vi "Input DMA Engine.vi"(10 "Parameters":variant, 11 "Process":refnum<class "Process.lvclass">) -> ()   [LabVIEW 2019, in "FPGA Addon Engine.lvlib"]
uses:
  FPGA Addon Engine.lvlib
  <vilib>/NI/NIVS Inline Async API/_VS Inline Async API/Process/Process.lvclass
  Types/DMA Input References.ctl
  <vilib>/NI VeriStand/Custom Device Waveform API/Multiple Waveforms Write (DBL)/Multiple Waveforms Write (DBL).lvclass
  Addon Shared/DMA Settings.ctl
  Addon Shared/Delacing Scheme.ctl
  Addon Shared/DMA Acquisition Mode.ctl
  Types/DMA Input Refs.ctl
  Addon Shared/Data Type.ctl
  <vilib>/NI/NIVS Inline Async API/_VS Inline Async API/Process/Process.lvclass/Process.ctl
  <vilib>/Platform/TimedLoop/XDataNode/timing_clust.ctl
  <vilib>/Platform/TimedLoop/XDataNode/nitl_modes.ctl
  <vilib>/Platform/TimedLoop/XDataNode/wakeup.ctl
  <vilib>/NI/NIVS Inline Async API/_Data Access Engine/Access Type Classes/Write/Write.lvclass/Write.ctl
  <vilib>/NI/NIVS Inline Async API/_Data Access Engine/Data Access Engine/Methods/Write.Data.vi
  <vilib>/NI/NIVS Inline Async API/_VS Inline Async API/Process/Data Member Access/Read Data Access.vi
  <vilib>/NI/NIVS Inline Async API/_Data Access Engine/Access Type Classes/Write/Write.ProcessData.vi
  <vilib>/NI/NIVS Inline Async API/_VS Inline Async API/Error Handling Process/SubVIs/Error.ConvertArray.vi
  <vilib>/NI/NIVS Inline Async API/_Data Access Engine/Access Type Classes/Write/Write.Buffer.vi
  <vilib>/NI/NIVS Inline Async API/_Data Access Engine/Access Type Classes/Write/Write.Commit.vi
  <vilib>/Utility/SystemLogging/Write to System Log.vi
  <vilib>/NI/NIVS Inline Async API/_Data Access Engine/Data Access Engine/Methods/Write.Lookup.vi
  <vilib>/FPGAPlugInAG/Dynamic/niLvFpga_Close_Dynamic.vi
  <vilib>/NI VeriStand/Custom Device Waveform API/Multiple Waveforms Write (DBL)/NI VeriStand - Close Multiple Waveforms Write Session (DBL).vi
  <vilib>/NI/NIVS Inline Async API/_Data Access Engine/Data Access Engine/Data Access Engine.lvclass
  <vilib>/Platform/TimedLoop/XDataNode/XDataNode.xnode
  <vilib>/rvi/interface/nirviCloseFPGA/nirviCloseFPGA.xnode
  <vilib>/NI VeriStand/Custom Device Waveform API/NI_VS Custom Device Waveform API.lvlib
  <vilib>/Platform/TimedLoop/XDataNode/XDNodeRunTimeDep.lvlib
  Addon Shared/FPGA Addon Shared.lvlib
panel:
  out "error out":errorcluster
  in  "error in (no error)":errorcluster
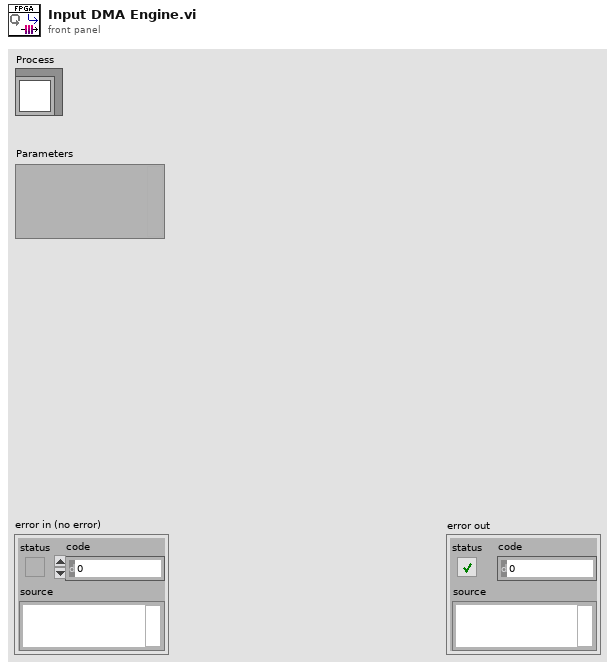
[diagram p1: front panel]
types:
  T1 = typedef "FPGA Addon Engine.lvlib/DMA Input References.ctl" = cluster{"Addon Name":string, "Waveform Ref":refnum<class "Multiple Waveforms Write (DBL).lvclass">, "DMA Name":string, "DMA Settings":T2, "Refs":T5}
  T2 = typedef "FPGA Addon Shared.lvlib/DMA Settings.ctl" = cluster{"Number of Channels":u8, "Delacing Scheme":T3, "Update Rate":u32, "dt":dbl, "Mode":T4, "Number of Samples":u32, "DMA Host Buffer":u32}
  T3 = typedef "FPGA Addon Shared.lvlib/Delacing Scheme.ctl" = enum8{"Interleaved", "Bitpacked"}
  T4 = typedef "FPGA Addon Shared.lvlib/DMA Acquisition Mode.ctl" = enum8{"Continuous", "Triggered Finite"}
  T5 = typedef "FPGA Addon Engine.lvlib/DMA Input Refs.ctl" = cluster{"Data Type":T6, "DMA_SGL":refnum<k20>, "DMA_U64":refnum<k20>, "DMA_I64":refnum<k20>, "DMA_FXP+/-32.8":refnum<k20>, "DMA_FXP+/-64.32":refnum<k20>, "DMA_U32":refnum<k20>, "DMA_U16":refnum<k20>, "DMA_U8":refnum<k20>, "DMA_I32":refnum<k20>, "DMA_I16":refnum<k20>, "DMA_I8":refnum<k20>, "DMA_FXP+/-32.16":refnum<k20>}
  T6 = typedef "FPGA Addon Shared.lvlib/Data Type.ctl" = enum8{"<Null>", "I8", "I16", "I32", "I64", "U8", "U16", "U32", "U64", "SGL", "Boolean", "Analog PWM In Settings", "Analog PWM In", "Digital PWM In Settings", "Digital PWM In", "Digital PWM Out", "Sine Out", "FXP+/-24.5", "FXP+/-16.5", "FXP+/-32.8", "FXP+/-64.32", "FXP+/-16.7", "FXP+/-20.5", "FXP+/-27.5", "FXP+/-32.16", "FXP +16.3", "FXP +18.3", "Digital Static In", "Digital Static Out", "Digital Static In Settings", "Digital WSS Out", "Quad Encoder Settings", "Quad Encoder In"}
  T7 = typedef "Data Access Engine.lvlib/Data Access Engine.lvclass/Write.DVR.ctl" = refnum<data-value>
  T8 = typedef "XDNodeRunTimeDep.lvlib/timing_clust.ctl" = cluster{"Expected End [f-1]":u64, "Actual End [f-1]":u64, "Finished Late? [f-1]":bool, "Expected End [i-1]":u64, "Actual End [i-1]":u64, "Finished Late? [i-1]":bool, "Expected Start [i]":u64, "Actual Start [i]":u64, "Expected Start [f]":u64, "Actual Start [f]":u64, "Source Name":string, "Structure Name":string, "Period":i64, "Deadline":i64, "Offset":i64, "Start":i64, "Priority":i32, "Timeout":i32, "Mode":T9, "Wakeup Reason":T10, "Error":errorcluster, "Source Type":string, "Secondary Source Type":string, "Global End Time":u64, "Global Start Time":u64, "Frame Duration":u64, "Iteration Duration":u64, "Assigned CPU":i32, "I/O Scan Engine Mode":u32}
  T9 = typedef "XDNodeRunTimeDep.lvlib/nitl_modes.ctl" = enum32{"No Change", "Process missed periods, maintain original phase", "Discard missed periods, maintain original phase", "Process missed periods, ignore original phase", "Discard missed periods, ignore original phase"}
  T10 = typedef "XDNodeRunTimeDep.lvlib/wakeup.ctl" = enum32{"Normal", "Aborted", "Asynchronous wakeup", "Timing source error", "Timed loop error", "Timeout"}
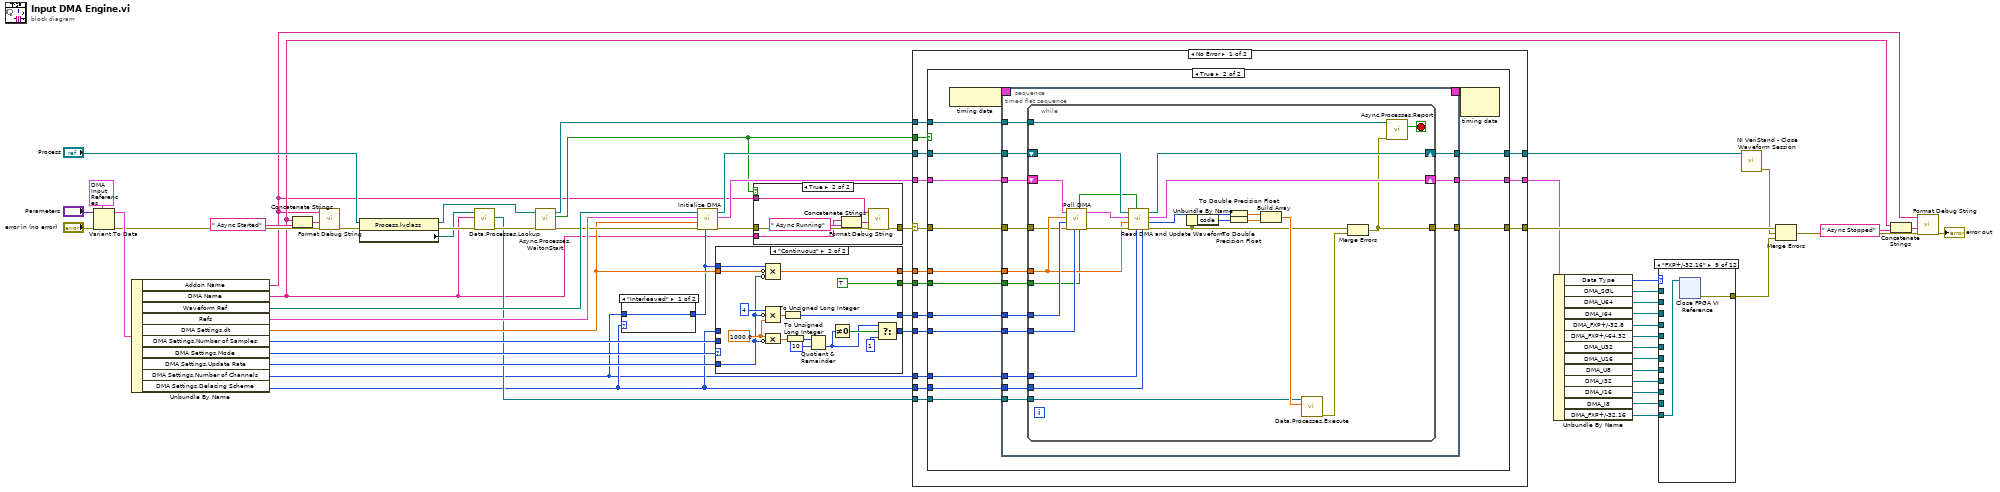
[diagram p0: block diagram]
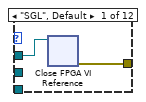
[diagram p2: hidden frame]
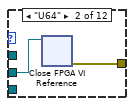
[diagram p3: hidden frame]
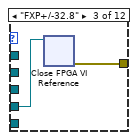
[diagram p4: hidden frame]
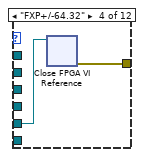
[diagram p5: hidden frame]
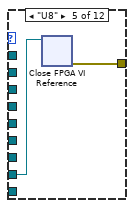
[diagram p6: hidden frame]
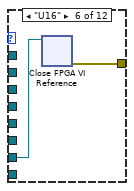
[diagram p7: hidden frame]
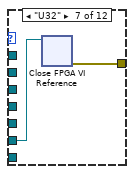
[diagram p8: hidden frame]
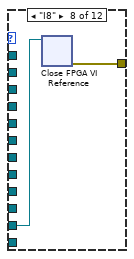
[diagram p9: hidden frame]
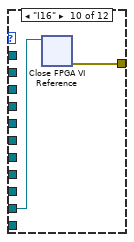
[diagram p10: hidden frame]
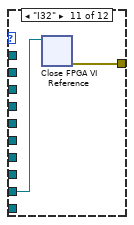
[diagram p11: hidden frame]
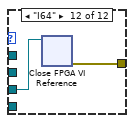
[diagram p12: hidden frame]
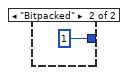
[diagram p13: hidden frame]
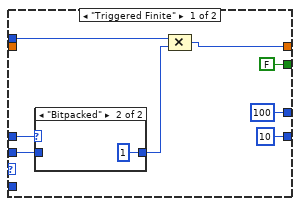
[diagram p14: hidden frame]
diagram:
  n1 = Variant To Data(error in="error in (no error)", type=T1 {"Addon Name"="", "Waveform Ref"=refnum, "DMA Name"="", "DMA Settings"={"Number of Channels"=0, "Delacing Scheme"=enum."Interleaved", "Update Rate"=0, "dt"=1000.0, "Mode"=enum."Continuous", "Number of Samples"=10000, "DMA Host Buffer"=5}, "Refs"={"Data Type"=enum."I32", "DMA_SGL"=refnum, "DMA_U64"=refnum, "DMA_I64"=refnum, "DMA_FXP+/-32.8"=refnum, "DMA_FXP+/-64.32"=refnum, "DMA_U32"=refnum, "DMA_U16"=refnum, "DMA_U8"=refnum, "DMA_I32"=refnum, "DMA_I16"=refnum, "DMA_I8"=refnum, "DMA_FXP+/-32.16"=refnum}} ("Parameters"), Variant="Parameters") -> (data=w30:T1, error out=w23:errorcluster)
  n2 = Unbundle By Name(w30) -> ("Addon Name"=w1:string, "DMA Name"=w2:string, "Waveform Ref"=w58:refnum<class "Multiple Waveforms Write (DBL).lvclass">, "Refs"=w51:T5, "DMA Settings.dt"=w44:dbl, "DMA Settings.Number of Samples"=w39:u32, "DMA Settings.Mode"=w40:T4, "DMA Settings.Update Rate"=w43:u32, "DMA Settings.Number of Channels"=w26:u8, "DMA Settings.Delacing Scheme"=w27:T3)
  n3 = Concatenate Strings(w2, " Async Started" ("string")) -> (w24:string)
  n4 = call "Format Debug String.vi"("error in (no error)"=w23, "State"=w24, "Name"=w1) -> ("error out"=w22:errorcluster)  [unwired: 8 in]
  n5 = property class="Process.lvclass"(reference="Process", error in=w22) -> (reference out=w37:refnum<class "Process.lvclass">, error out=w36:errorcluster, "Data Member Access:Data Access"=w34:refnum<class "Data Access Engine.lvclass">)
  n6 = call-poly <vilib>:"Data.Processes.Lookup.vi"("error in (no error)"=w36, "Name"=w2, "Data Access API in"=w34) -> ("error out"=w35:errorcluster, "Ref"=w33:T7)  [unwired: 5 in, 2 out]
  n7 = call <vilib>:"Async.Processes.WaitonStart.vi"("error in (no error)"=w35, "Process"=w37) -> ("error out"=w49:errorcluster, "Execute"=w50:bool, "Process out"=w32:refnum<class "Process.lvclass">)  [unwired: 7 in]
  n8 = case shown="\"Interleaved\"" w27 {
    tunnel: [w59 u8 1 ("Number of Channels")] -> w28
    tunnel: w26 -> [w59 _]
    frame "Interleaved" {
    }
    frame "Bitpacked" {
    }
  }
  n9 = call "Initialize DMA.vi"("Number of Channels"=w28, "error in (no error)"=w49, "dt"=w44, "Refs"=w51, "Multiple Waveforms Write (DBL) in"=w58) -> ("error out"=w48:errorcluster, "Refs"=w56:T5, "Multiple Waveforms Write (DBL) out"=w57:refnum<class "Multiple Waveforms Write (DBL).lvclass">)  [unwired: 4 in]
  n10 = case shown="\"Continuous\"" w40 {
    tunnel: [u32 10 ("f") w79] -> w46
    tunnel: [u32 100 w76] -> w45
    tunnel: w28 -> [w68 w75]
    tunnel: w44 -> [_ w74]
    tunnel: w43 -> [_ w73]
    tunnel: [w67 w72] -> w42
    tunnel: [FALSE TRUE] -> w41
    tunnel: w39 -> [w61 _]
    tunnel: w27 -> [w63 _]
    frame "Triggered Finite" {
      n11 = case shown="\"Bitpacked\"" w63 {
        tunnel: [w69 u32 1 ("Number of Samples")] -> w62
        tunnel: w61 -> [w69 _]
        frame "Interleaved" {
        }
        frame "Bitpacked" {
        }
      }
      n12 = Compound Arithmetic op=MULTIPLY(w68, w62) -> (w67:u32)
    }
    frame "Continuous" {
      w77 = 1000.0 ("y")
      n13 = Compound Arithmetic op=MULTIPLY(w75, invert w74, invert w73) -> (w72:dbl)
      n14 = Compound Arithmetic op=MULTIPLY(u32 4 ("value"), invert w73, w77) -> (w78:dbl)
      n15 = Compound Arithmetic op=MULTIPLY(w77, invert w73) -> (w81:dbl)
      n16 = To Unsigned Long Integer(number=w78) -> (unsigned 32bit integer=w76:u32)
      n17 = To Unsigned Long Integer(number=w81) -> (unsigned 32bit integer=w82:u32)
      n18 = Quotient & Remainder(x=w82, y=u32 10) -> (floor(x/y)=w80:u32)  [unwired: 1 out]
      n19 = Not Equal To 0?(x=w80) -> (x != 0?=w85:bool)
      n20 = Select(t=w80, s=w85, f=u32 1) -> (s? t:f=w79:u32)
    }
  }
  n21 = case shown="True" w50 {
    tunnel: w2 -> [_ w89]
    tunnel: w48 -> [w87 w91]
    tunnel: [w87 w90] -> w47
    tunnel: w1 -> [_ w88]
    frame False {
    }
    frame True {
      n22 = Concatenate Strings(w89, " Async Running" ("string")) -> (w92:string)
      n23 = call "Format Debug String.vi"("error in (no error)"=w91, "State"=w92, "Name"=w88) -> ("error out"=w90:errorcluster)  [unwired: 8 in]
    }
  }
  n24 = case shown="No Error" w47 {
    selector: w47 -> [w100 w187]
    tunnel: w57 -> [w108 w186]
    tunnel: w56 -> [w107 w185]
    tunnel: w42 -> [w106 _]
    tunnel: w26 -> [w105 _]
    tunnel: [w104 w186] -> w55
    tunnel: [w103 w187] -> w54
    tunnel: w45 -> [w102 _]
    tunnel: w32 -> [w101 _]
    tunnel: w50 -> [w99 _]
    tunnel: w46 -> [w98 _]
    tunnel: [w97 w185] -> w52
    tunnel: w27 -> [w96 _]
    tunnel: w33 -> [w95 _]
    tunnel: w41 -> [w94 _]
    frame No Error {
      n25 = case shown="True" w99 {
        tunnel: w108 -> [w111 w127]
        tunnel: w107 -> [w109 w126]
        tunnel: w106 -> [_ w125]
        tunnel: w105 -> [_ w124]
        tunnel: [w111 w123] -> w104
        tunnel: [w110 w116] -> w103
        tunnel: w102 -> [_ w122]
        tunnel: w101 -> [_ w121]
        tunnel: w100 -> [w110 w115]
        tunnel: w98 -> [_ w120]
        tunnel: [w109 w119] -> w97
        tunnel: w96 -> [_ w118]
        tunnel: w95 -> [_ w117]
        tunnel: w94 -> [_ w114]
        frame False {
        }
        frame True {
          n26 = node-c288() -> (w113:T8)
          n27 = timed-sequence {
            timing: w113 -> [_]
            timing-out: [_] -> w112
            tunnel: w127 -> [w141]
            tunnel: w126 -> [w140]
            tunnel: w125 -> [w139]
            tunnel: w124 -> [w138]
            tunnel: [w137] -> w123
            tunnel: w122 -> [w136]
            tunnel: w121 -> [w135]
            tunnel: w120 -> [w134]
            tunnel: [w133] -> w119
            tunnel: w118 -> [w132]
            tunnel: w117 -> [w131]
            tunnel: [w130] -> w116
            tunnel: w115 -> [w129]
            tunnel: w114 -> [w128]
            n28 = timed-flat-sequence {
              tunnel: w141 -> [w155]
              tunnel: w140 -> [w154]
              tunnel: w139 -> [w153]
              tunnel: w138 -> [w152]
              tunnel: [w151] -> w137
              tunnel: w136 -> [w150]
              tunnel: w135 -> [w149]
              tunnel: w134 -> [w148]
              tunnel: [w147] -> w133
              tunnel: w132 -> [w146]
              tunnel: w131 -> [w145]
              tunnel: [w144] -> w130
              tunnel: w129 -> [w143]
              tunnel: w128 -> [w142]
              n29 = while {
                tunnel: w150 -> [w178]
                tunnel: w153 -> [w166]
                tunnel: w152 -> [w165]
                tunnel: w149 -> [w176]
                tunnel: w148 -> [w174]
                tunnel: w146 -> [w164]
                tunnel: w145 -> [w171]
                shift-right: [w168] -> w147
                shift-left: w154 -> [w179]
                shift-right: [w177] -> w151
                shift-left: w155 -> [w180]
                tunnel: [w162] -> w144
                tunnel: w143 -> [w161]
                tunnel: w142 -> [w159]
                stop <- w158 stop-if-true
                n30 = call "Poll DMA.vi"("Timeout is Error?"=w159, "Wait (ms)"=w174, "error in (no error)"=w161, "Timeout (ms)"=w178, "Total Samples to Read"=w166, "Refs"=w179) -> ("error out"=w175:errorcluster, "Refs"=w167:T5, "Timeout?"=w160:bool)  [unwired: 3 in]
                n31 = call "Read DMA and Update Waveform.vi"("Delacing Scheme"=w164, "Number of Channels"=w165, "Timeout?"=w160, "error in (no error)"=w175, "Total Samples"=w166, "Refs in"=w167, "Multiple Waveforms Write (DBL) in"=w180) -> ("error out"=w163:errorcluster, "Elements Remaining"=w169:u32, "Refs in"=w168:T5, "Multiple Waveforms Write (DBL) out"=w177:refnum<class "Multiple Waveforms Write (DBL).lvclass">)  [unwired: 1 in]
                n32 = Unbundle By Name(w163) -> ("code"=w173:i32)
                n33 = To Double Precision Float(number=w169) -> (double precision float=w156:dbl)
                n34 = To Double Precision Float(number=w173) -> (double precision float=w157:dbl)
                n35 = Build Array(w156, w157) -> (w172:dbl[])
                n36 = call-poly <vilib>:"Data.Processes.Execute.vi"("Values"=w172, "Ref"=w171) -> ("error out"=w170:errorcluster)  [unwired: 9 in]
                n37 = Merge Errors(w163, w170) -> (w162:errorcluster)
                n38 = call <vilib>:"Async.Processes.Report.vi"("Error"=w162, "Process in"=w176) -> ("Stop"=w158:bool)  [unwired: 8 in, 1 out]
              }
            }
          }
          n39 = node-c288(w112) -> ()  [unwired: 1 out]
        }
      }
    }
    frame Error {
    }
  }
  n40 = Unbundle By Name(w52) -> ("Data Type"=w20:T6, "DMA_SGL"=w19:refnum<k20>, "DMA_U64"=w18:refnum<k20>, "DMA_I64"=w16:refnum<k20>, "DMA_FXP+/-32.8"=w15:refnum<k20>, "DMA_FXP+/-64.32"=w14:refnum<k20>, "DMA_U32"=w13:refnum<k20>, "DMA_U16"=w12:refnum<k20>, "DMA_U8"=w11:refnum<k20>, "DMA_I32"=w10:refnum<k20>, "DMA_I16"=w9:refnum<k20>, "DMA_I8"=w8:refnum<k20>, "DMA_FXP+/-32.16"=w7:refnum<k20>)
  n41 = case shown="\"FXP+/-32.16\"" w20 {
    tunnel: [w189 w191 w193 w195 w197 w199 w201 w203 w205 w207 w209 w211] -> w17
    tunnel: w19 -> [w188 _ _ _ _ _ _ _ _ _ _ _]
    tunnel: w18 -> [_ w190 _ _ _ _ _ _ _ _ _ _]
    tunnel: w16 -> [_ _ _ _ _ _ _ _ _ _ _ w210]
    tunnel: w15 -> [_ _ w192 _ _ _ _ _ _ _ _ _]
    tunnel: w14 -> [_ _ _ w194 _ _ _ _ _ _ _ _]
    tunnel: w13 -> [_ _ _ _ _ _ w200 _ _ _ _ _]
    tunnel: w12 -> [_ _ _ _ _ w198 _ _ _ _ _ _]
    tunnel: w11 -> [_ _ _ _ w196 _ _ _ _ _ _ _]
    tunnel: w10 -> [_ _ _ _ _ _ _ _ _ _ w208 _]
    tunnel: w9 -> [_ _ _ _ _ _ _ _ _ w206 _ _]
    tunnel: w8 -> [_ _ _ _ _ _ _ w202 _ _ _ _]
    tunnel: w7 -> [_ _ _ _ _ _ _ _ w204 _ _ _]
    frame "SGL", Default {
      n42 = xnode "Close FPGA VI Reference"("FPGA VI Reference In"=w188) -> ("error out"=w189:errorcluster)  [unwired: 1 in]
    }
    frame "U64" {
      n43 = xnode "Close FPGA VI Reference"("FPGA VI Reference In"=w190) -> ("error out"=w191:errorcluster)  [unwired: 1 in]
    }
    frame "FXP+/-32.8" {
      n44 = xnode "Close FPGA VI Reference"("FPGA VI Reference In"=w192) -> ("error out"=w193:errorcluster)  [unwired: 1 in]
    }
    frame "FXP+/-64.32" {
      n45 = xnode "Close FPGA VI Reference"("FPGA VI Reference In"=w194) -> ("error out"=w195:errorcluster)  [unwired: 1 in]
    }
    frame "U8" {
      n46 = xnode "Close FPGA VI Reference"("FPGA VI Reference In"=w196) -> ("error out"=w197:errorcluster)  [unwired: 1 in]
    }
    frame "U16" {
      n47 = xnode "Close FPGA VI Reference"("FPGA VI Reference In"=w198) -> ("error out"=w199:errorcluster)  [unwired: 1 in]
    }
    frame "U32" {
      n48 = xnode "Close FPGA VI Reference"("FPGA VI Reference In"=w200) -> ("error out"=w201:errorcluster)  [unwired: 1 in]
    }
    frame "I8" {
      n49 = xnode "Close FPGA VI Reference"("FPGA VI Reference In"=w202) -> ("error out"=w203:errorcluster)  [unwired: 1 in]
    }
    frame "FXP+/-32.16" {
      n50 = xnode "Close FPGA VI Reference"("FPGA VI Reference In"=w204) -> ("error out"=w205:errorcluster)  [unwired: 1 in]
    }
    frame "I16" {
      n51 = xnode "Close FPGA VI Reference"("FPGA VI Reference In"=w206) -> ("error out"=w207:errorcluster)  [unwired: 1 in]
    }
    frame "I32" {
      n52 = xnode "Close FPGA VI Reference"("FPGA VI Reference In"=w208) -> ("error out"=w209:errorcluster)  [unwired: 1 in]
    }
    frame "I64" {
      n53 = xnode "Close FPGA VI Reference"("FPGA VI Reference In"=w210) -> ("error out"=w211:errorcluster)  [unwired: 1 in]
    }
  }
  n54 = call-poly <vilib>:"NI VeriStand - Close Waveform Session.vi"("Multiple Waveforms Write Session (DBL)"=w55) -> ("error out"=w21:errorcluster)  [unwired: 10 in]
  n55 = Merge Errors(w54, w21, w17) -> (w4:errorcluster)
  n56 = Concatenate Strings(w2, " Async Stopped" ("string")) -> (w5:string)
  n57 = call "Format Debug String.vi"("error in (no error)"=w4, "State"=w5, "Name"=w1) -> ("error out"=→"error out":errorcluster)  [unwired: 8 in]
